vi "ReadFromTextFile.vi"() -> ()   [LabVIEW 2022 SP3]
panel:
  in  "stop":bool
  out "output waveform":waveform(dbl)
  out "Waveform Chart":dbl(graph)
  out "offset (in bytes)":i64
  out "Search Pattern":string
  in  "Separator":string="."
  in  "Delimiter":string="\t"
  in  "Skip Lines":i32=21
  in  "Path":path=path "C:/Users/LAV-UFSC/Desktop/acc_time/Previous Data/handlebar_acc1_run1.txt"
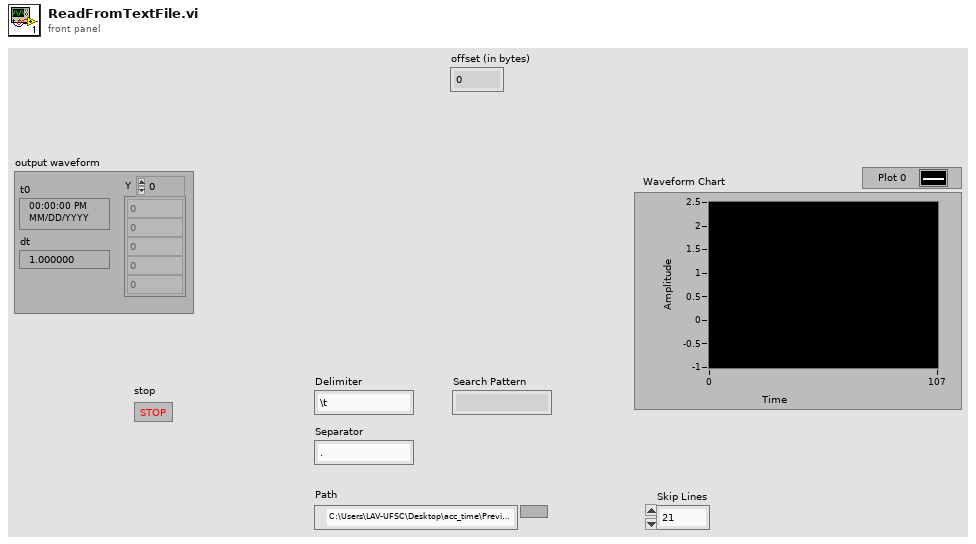
[diagram p1: front panel]
types:
  T1 = enum16{"open", "replace", "create", "open or create", "replace or create", "replace or create with confirmation"}
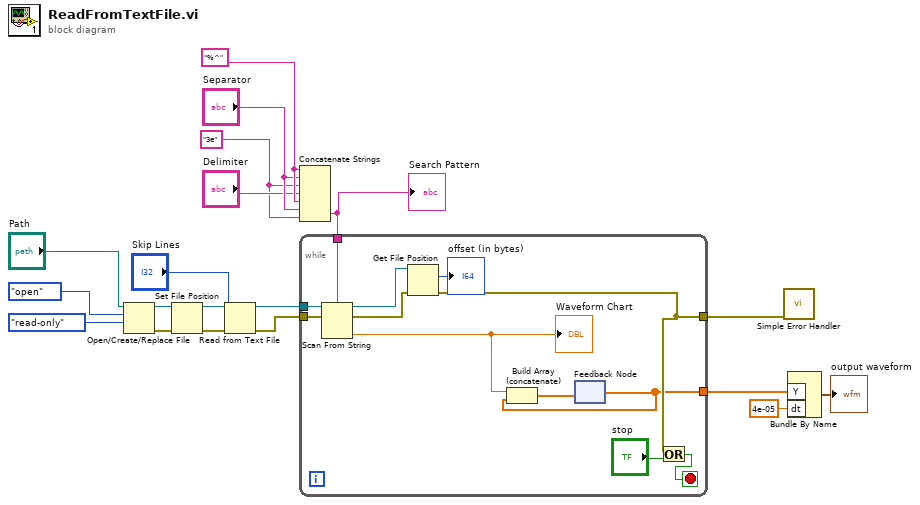
[diagram p0: block diagram]
diagram:
  w5 = "3e" ("string")
  w12 = "%^" ("format string")
  n1 = Open/Create/Replace File(file path (use dialog)="Path", operation (0:open)=T1."open", access (0:read/write)=enum16{"read/write", "read-only", "write-only"}."read-only") -> (refnum out=w7:refnum<file>, error out=w16:errorcluster)  [unwired: 3 in, 1 out]
  n2 = Set File Position(refnum=w7, error in=w16) -> (refnum out=w8:refnum<file>, error out=w17:errorcluster)  [unwired: 2 in]
  n3 = Read from Text File(file (use dialog)=w8, count="Skip Lines") -> (refnum out=w9:refnum<file>)  [unwired: 2 in, 3 out]
  n4 = Concatenate Strings(w12, "Separator", w5, "Delimiter", w12, "Separator", w5) -> (w6:string)
  "Search Pattern" <- w6
  n5 = while {
    tunnel: w17 -> [w30]
    tunnel: w9 -> [w29]
    tunnel: w6 -> [w28]
    tunnel: [w23] -> w4
    tunnel: [w19] -> w3
    stop <- w21 stop-if-true
    n6 = Scan From String(w28, w29, w30) -> (w27:refnum<file>, w26:errorcluster, output 2=w24:dbl)  [unwired: 3 in]
    "Waveform Chart" <- w24
    n7 = Get File Position(4:w26, 7:w27) -> (0:w23:errorcluster, 2:→"offset (in bytes)":i64)  [unwired: 1 out]
    n8 = feedback #1() -> (w19:dbl[])  [unwired: 1 in]
    n9 = Build Array (concatenate)(w24, w19) -> (w20:dbl[])
    n10 = feedback-in #1(w20) -> ()
    n11 = Or(x=w23, y="stop") -> (x .or. y?=w21:bool)
  }
  n12 = call <vilib>:"Simple Error Handler.vi"("error in (no error)"=w4) -> ()  [unwired: 4 in, 5 out]
  n13 = Bundle By Name("Y"=w3, "dt"=4e-05) -> (→"output waveform":waveform(dbl))  [unwired: 1 in]
